vi "Millisecond Time Delay.vi"(5 "milliseconds to wait":u32, 7 "error in (no error)":errorcluster) -> (1 "error out":errorcluster)   [LabVIEW 2020, in "Framework Test Support.lvlib"]
doc: "Waits specified number of milliseconds if no upstreams error."
uses:
  Framework Test Support.lvlib
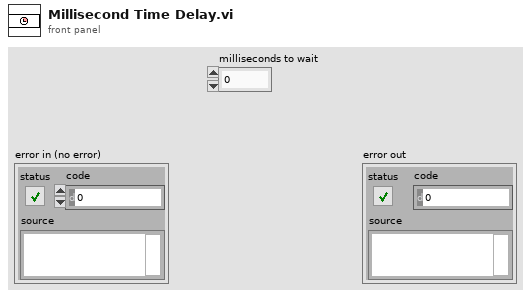
[diagram p1: front panel]
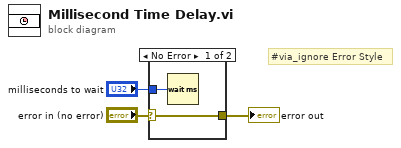
[diagram p0: block diagram]
diagram:
  # "#via_ignore Error Style"
  n1 = case shown="No Error" "error in (no error)" {
    selector: "error in (no error)" -> [w4 w6]
    tunnel: "milliseconds to wait" -> [w5 _]
    tunnel: [w4 w6] -> w2
    frame No Error {
      n2 = Wait (ms)(milliseconds to wait=w5) -> ()  [unwired: 1 out]
    }
    frame Error {
    }
  }
  "error out" <- w2
